vi "Drive_Motor_Speed_Test.vi"() -> ()   [LabVIEW 2020]
panel:
  out "Right Speed":cluster{"RightSpeed":dbl, "Left Dmd":dbl}(graph)
  out "Left Speed":cluster{"Left Dmd":dbl, "LeftSpeed":dbl}(graph)
  out "Left Spd":dbl
  out "Right Spd":dbl
  in  "Right Dmd":dbl(slide) scale=-10.0..10.0
  in  "Left Dmd":dbl(slide) scale=-10.0..10.0
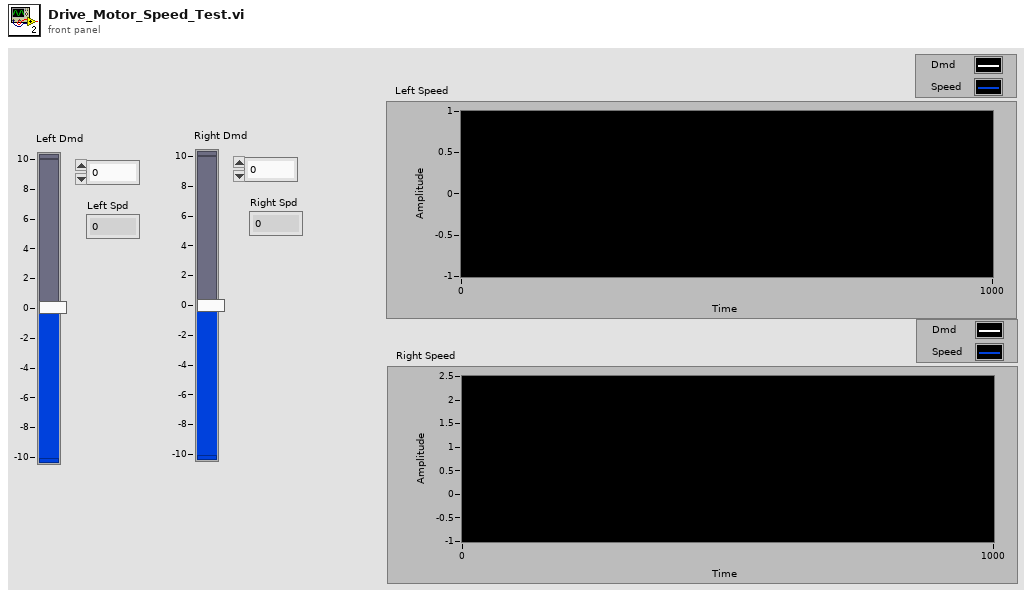
[diagram p1: front panel]
types:
  T1 = typedef "WPI_RobotDriveDevRef.ctl" = cluster{"DevStatus":errorcluster, "Motors[]":T2[], "Square Inputs":bool, "Max Output":dbl}
  T2 = typedef "WPI_MotorControlDeviceRef.ctl" = cluster{"DeviceStatus":errorcluster, "Type":T3, "PWM":cluster{"PWM Channel":T4, "DeadBand":T5}, "CAN":cluster{"Device Number":u8, "SetOutput VI Ref":variant, "GetOutput VI Ref":variant, "Enable VI Ref":variant, "Disable VI Ref":variant, "Data":variant}, "Invert":bool, "DIO PWM":cluster{"PWM \"Enable\" Channel":T4, "DIOChannel":T6, "PWM Rate":dbl}}
  T3 = typedef "WPI_MotorControlType.ctl" = enum16{"PWM", "CAN", "DIO PWM"}
  T4 = typedef "FPGA_DIOPWMChannel.ctl" = enum8{"PWM 0", "PWM 1", "PWM 2", "PWM 3", "PWM 4", "PWM 5", "PWM 6", "PWM 7", "PWM 8", "PWM 9", "PWM MXP 0", "PWM MXP 1", "PWM MXP 2", "PWM MXP 3", "PWM MXP 4", "PWM MXP 5", "PWM MXP 6", "PWM MXP 7", "PWM MXP 8", "PWM MXP 9", "Invalid"}
  T5 = typedef "WPI_PWMDeadband.ctl" = cluster{"Name":string, "maxPositivePwm":i32, "minPositivePwm":i32, "centerPwm":i32, "maxNegativePwm":i32, "minNegativePwm":i32, "angularRange":u16}
  T6 = typedef "FPGA_DIOChannel.ctl" = enum8{"DIO 0", "DIO 1", "DIO 2", "DIO 3", "DIO 4", "DIO 5", "DIO 6", "DIO 7", "DIO 8", "DIO 9", "DIO MXP 0", "DIO MXP 1", "DIO MXP 2", "DIO MXP 3", "DIO MXP 4", "DIO MXP 5", "DIO MXP 6", "DIO MXP 7", "DIO MXP 8", "DIO MXP 9", "DIO MXP 10", "DIO MXP 11", "DIO MXP 12", "DIO MXP 13", "DIO MXP 14", "DIO MXP 15", "SPI Port CS1", "SPI Port CS2", "SPI Port CS3", "SPI Port MISO", "SPI Port MOSI", "Invalid"}
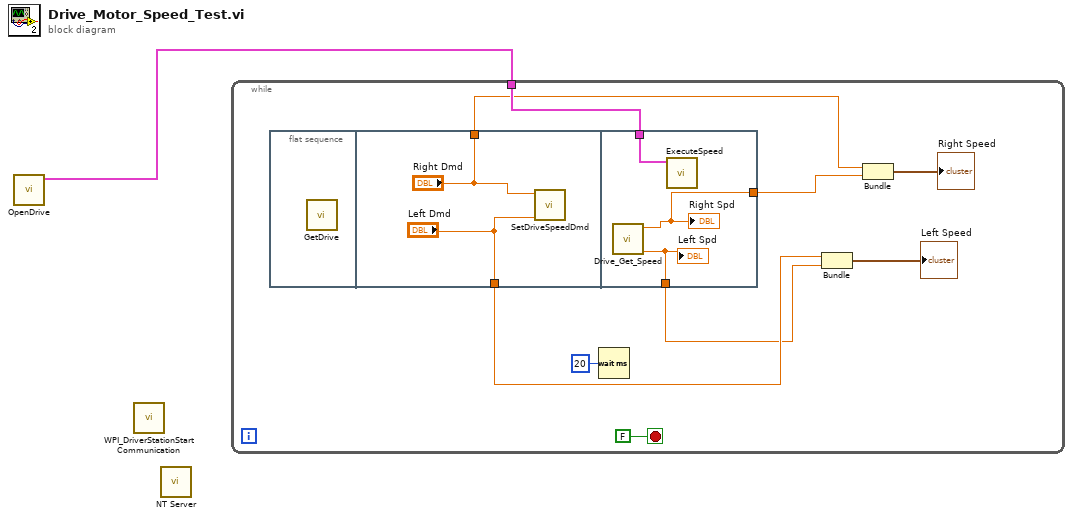
[diagram p0: block diagram]
diagram:
  n1 = call "OpenDrive.vi"() -> ("RobotDriveDevRef"=w1:T1)  [unwired: 11 in]
  n2 = call <vilib>:"WPI_DriverStationStart Communication.vi"() -> ()  [unwired: 12 in]
  n3 = call <vilib>:"NT Server.vi"() -> ()  [unwired: 12 in]
  n4 = while {
    tunnel: w1 -> [w8]
    stop <- FALSE stop-if-true
    n5 = flat-sequence {
      tunnel: ["Left Dmd"] -> w7
      tunnel: ["Right Dmd"] -> w2
      tunnel: w8 -> [w15]
      tunnel: [w14] -> w6
      tunnel: [w13] -> w3
      frame #0 {
        n6 = call "GetDrive.vi"() -> ()  [unwired: 11 in, 1 out]
      }
      frame #1 {
        n7 = call "SetDriveSpeedDmd.vi"("LeftSpeedInput"="Left Dmd", "RightSpeedInput"="Right Dmd") -> ()  [unwired: 10 in]
      }
      frame #2 {
        n8 = call "Drive_Get_Speed.vi"() -> ("LeftSpeed"=w14:dbl, "RightSpeed"=w13:dbl)  [unwired: 10 in]
        "Left Spd" <- w14
        "Right Spd" <- w13
        n9 = call "ExecuteSpeed.vi"("RobotDriveDevRef"=w15) -> ()  [unwired: 10 in, 1 out]
      }
    }
    n10 = Wait (ms)(milliseconds to wait=u32 20) -> ()  [unwired: 1 out]
    n11 = Bundle("Left Dmd"=w7, "LeftSpeed"=w6) -> (→"Left Speed":cluster{"Left Dmd":dbl, "LeftSpeed":dbl})  [unwired: 1 in]
    n12 = Bundle("Right Dmd"=w2, "RightSpeed"=w3) -> (→"Right Speed":cluster{"Right Dmd":dbl, "RightSpeed":dbl})  [unwired: 1 in]
  }
